vi "150203-Counter-SinglePulseOutput.vi"(8 "error in":errorcluster, 10 "Pulse Duration":dbl=150.0 format="%.6f") -> (0 "error out 2":errorcluster)   [LabVIEW 2013]
doc: "This example demonstrates how to generate a single pulse using a counter output. \n\nThe single pulse may be triggered once or repeatedly from an external source."
uses:
  <vilib>/Utility/error.llb/DialogType.ctl
  <vilib>/DAQmx/create/channels.llb/DAQmx Create Channel (CO-Pulse Generation-Time).vi
  <vilib>/DAQmx/configure/trigger.llb/DAQmx Start Trigger (Digital Edge).vi
  <resource>/objmgr/daqmx.rc
panel:
  in  "Output Terminal":tag="/Dev4/PFI20"
  in  "Trigger Type":enum32{"No Trigger", "Digital Start"}(tab)
  in  "Retriggerable":bool
  in  "Edge":i32(ring)=10280 items=["Rising"=10280, "Falling"=10171]
  in  "Digital Trigger Source":tag
  in  "Stop":bool
  in  "Counter":tag="Dev4/ctr4"
  # "Channel Settings"
  # "Trigger Settings"
  # "To configure and use a trigger you must have the necessary tab selected above."
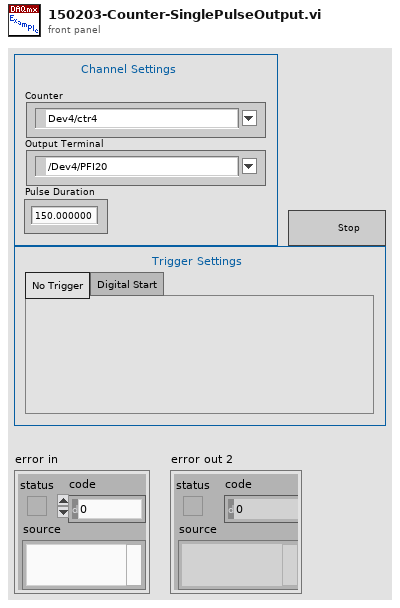
[diagram p1: front panel]
types:
  T1 = typedef "DialogType.ctl" = u16
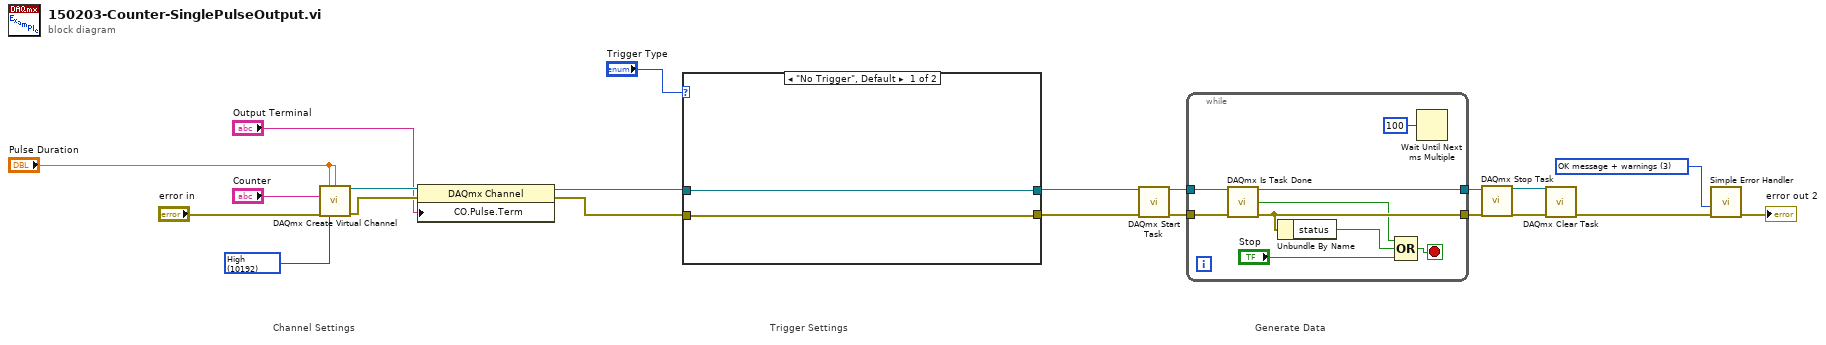
[diagram p0: block diagram]
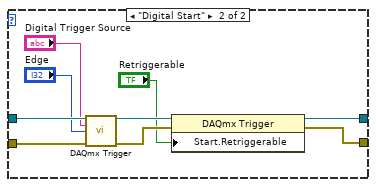
[diagram p2: hidden frame]
diagram:
  w1 = 10192 items=["High"=10192, "Low"=10214] ("idle state")
  w4 = T1 3 items=["no dialog", "OK message", "continue or stop message", "OK message + warnings", "continue/stop + warnings"] ("type of dialog (OK msg:1)")
  # "Generate Data"
  # "Trigger Settings"
  # "Channel Settings"
  n1 = call-poly <vilib>:"DAQmx Create Virtual Channel.vi"("high time"="Pulse Duration", "low time"="Pulse Duration", "counter"="Counter", "error in"="error in", "idle state"=w1) -> ("task out"=w14:refnum<k21>, "error out"=w13:errorcluster)  [unwired: 9 in]
  n2 = property class="DAQmx Channel"(reference=w14, error in=w13, "CO.Pulse.Term"="Output Terminal") -> (reference out=w10:refnum<k21>, error out=w11:errorcluster)
  n3 = case shown="\"No Trigger\", Default" "Trigger Type" {
    tunnel: w10 -> [w23 w32]
    tunnel: w11 -> [w22 w31]
    tunnel: [w23 w28] -> w15
    tunnel: [w22 w27] -> w16
    frame "No Trigger", Default {
    }
    frame "Digital Start" {
      n4 = call-poly <vilib>:"DAQmx Trigger.vi"("task/channels in"=w32, "source"="Digital Trigger Source", "edge"="Edge", "error in"=w31) -> ("task out"=w25:refnum<k21>, "error out"=w26:errorcluster)  [unwired: 10 in]
      n5 = property class="DAQmx Trigger"(reference=w25, error in=w26, "Start.Retriggerable"="Retriggerable") -> (reference out=w28:refnum<k21>, error out=w27:errorcluster)
    }
  }
  n6 = call <vilib>:"DAQmx Start Task.vi"("task/channels in"=w15, "error in"=w16) -> ("task out"=w21:refnum<k21>, "error out"=w20:errorcluster)  [unwired: 12 in]
  n7 = while {
    tunnel: w21 -> [w41]
    tunnel: w20 -> [w40]
    tunnel: [w37] -> w7
    tunnel: [w38] -> w8
    stop <- w39 stop-if-true
    n8 = call <vilib>:"DAQmx Is Task Done.vi"("task/channels in"=w41, "error in"=w40) -> ("task out"=w38:refnum<k21>, "task done?"=w33:bool, "error out"=w37:errorcluster)  [unwired: 11 in]
    n9 = Unbundle By Name(w37) -> ("status"=w36:bool)
    n10 = Compound Arithmetic op=OR(w33, w36, "Stop") -> (w39:bool)
    n11 = Wait Until Next ms Multiple(millisecond multiple=u32 100) -> ()  [unwired: 1 out]
  }
  n12 = call <vilib>:"DAQmx Stop Task.vi"("task/channels in"=w8, "error in"=w7) -> ("task out"=w6:refnum<k21>, "error out"=w5:errorcluster)  [unwired: 12 in]
  n13 = call <vilib>:"DAQmx Clear Task.vi"("task in"=w6, "error in"=w5) -> ("error out"=w19:errorcluster)  [unwired: 13 in]
  n14 = call <vilib>:"Simple Error Handler.vi"("type of dialog (OK msg:1)"=w4, "error in (no error)"=w19) -> ("error out"=→"error out 2":errorcluster)  [unwired: 3 in, 4 out]
